vi "Actor Core.vi"(8 "error in":errorcluster, 11 "Rigol DG822 UI in":refnum<class "Rigol DG822 UI.lvclass">) -> (0 "error out":errorcluster, 3 "Actor out":refnum<class "Actor.lvclass">)   [LabVIEW 2021, in "Rigol DG822 UI.lvlib" / "Rigol DG822 UI.lvclass"]
uses:
  Rigol DG822 UI.lvclass
  General/Files/lvlibp/Actor Framework.lvlibp/1abvi3w/vi.lib/ActorFramework/Actor/Actor.lvclass
  D:/LabVIEW/General/Files/lvlibp/Actor Framework.lvlibp/1abvi3w/vi.lib/ActorFramework/Actor/Actor.lvclass
  D:/LabVIEW/General/Files/lvlibp/Actors.lvlibp/Actors/Actors/Actors.lvclass
  lib/controls.llb/DataCluster.ctl
  lib/controls.llb/String Indicators Cluster.ctl
  lib/controls.llb/FT Controls Cluster.ctl
  Rigol DG822 UI.lvclass/Rigol DG822 UI.ctl
  <vilib>/Utility/miscctls.llb/LVPointTypeDef.ctl
  lib/controls.llb/WaveformExtCall.ctl
  lib/controls.llb/WaveformSelector.ctl
  lib/controls.llb/RDG822ExtCall.ctl
  lib/controls.llb/AllWaveformDataCluster.ctl
  <userlib>/_MGI/Application Control/MGI VI Reference/MGI Current VI's Reference.vi
  <userlib>/_MGI/Timing/MGI Wait/MGI Wait (U32).vi
  General/Files/lvlibp/Actors.lvlibp/Actors/Actors/Actors.lvclass
  General/Files/lvlibp/Tools.lvlibp
panel:
  out "Data":T1={"Freq"={"Freq"=1.0, "FreqUnit"=enum."kHz", "FreqUnitPrcs"=9.0}, "Period"={"Period"=1.0, "PeriodUnit"=enum."ms", "PeriodUnitPrcs"=7.0}, "Ampl"={"Ampl"=5.0, "AmplUnit"=enum."Vpp", "AmplUnitPrcs"=4.0}, "HighL"={"HighL"=2.5, "HighLUnit"=enum."V", "HighLUnitPrcs"=4.0}, "Offset"={"Offset"=0.0, "OffsetUnit"=enum."Vdc", "OffsetUnitPrcs"=4.0}, "LowL"={"LowL"=-2.5, "LowLUnit"=enum."V", "LowLUnitPrcs"=4.0}, "Phase"={"Phase"=0.0, "PhaseUnit"=enum."°", "PhaseUnitPrcs"=3.0}, "Duty"={"Duty"=50.0, "DutyUnit"=enum."%", "DutyUnitPrcs"=3.0}, "Width"={"Width"=500.0, "WidthUnit"=enum."us", "WidthUnitPrcs"=4.0}, "RisEdge"={"RisEdge"=10.0, "RisEdgeUnit"=enum."ns", "RisEdgeUnitPrcs"=1.0}, "FallEdge"={"FallEdge"=10.0, "FallEdgeUnit"=enum."ns", "FallEdgeUnitPrcs"=1.0}} {"RisEdge"."RisEdge" format="%.1f"; "RisEdge"."RisEdgeUnitPrcs" format="%#_1g"; "FallEdge"."FallEdge" format="%.1f"; "FallEdge"."FallEdgeUnitPrcs" format="%#_1g"; "Width"."Width" format="%.4g"; "Width"."WidthUnitPrcs" format="%#_1g"; "Duty"."Duty" format="%.3g"; "Duty"."DutyUnitPrcs" format="%#_1g"; "Phase"."Phase" format="%.3g"; "Phase"."PhaseUnitPrcs" format="%#_1g"; "LowL"."LowL" format="%.4g"; "LowL"."LowLUnitPrcs" format="%#_1g"; "Offset"."Offset" format="%.4g"; "Offset"."OffsetUnitPrcs" format="%#_1g"; "HighL"."HighL" format="%.4g"; "HighL"."HighLUnitPrcs" format="%#_1g"; "Ampl"."Ampl" format="%.4g"; "Ampl"."AmplUnitPrcs" format="%#_1g"; "Period"."Period" format="%.7g"; "Period"."PeriodUnitPrcs" format="%#_1g"; "Freq"."FreqUnitPrcs" format="%#_1g"; "Freq"."Freq" format="%.9g"}
  in  "Out2":bool
  in  "Out1":bool
  in  "Home":bool
  in  "Main Tab":enum32{"Menu", "Wf Conf", "UpdScreen"}(tab)=enum."Wf Conf"
  in  "Wf Selector":T2(radio)=enum."Sine"
  out "Screen":picture
  in  "Menu":bool
  # "УБРАТЬ SINE ИЗ COERCE VALUE"
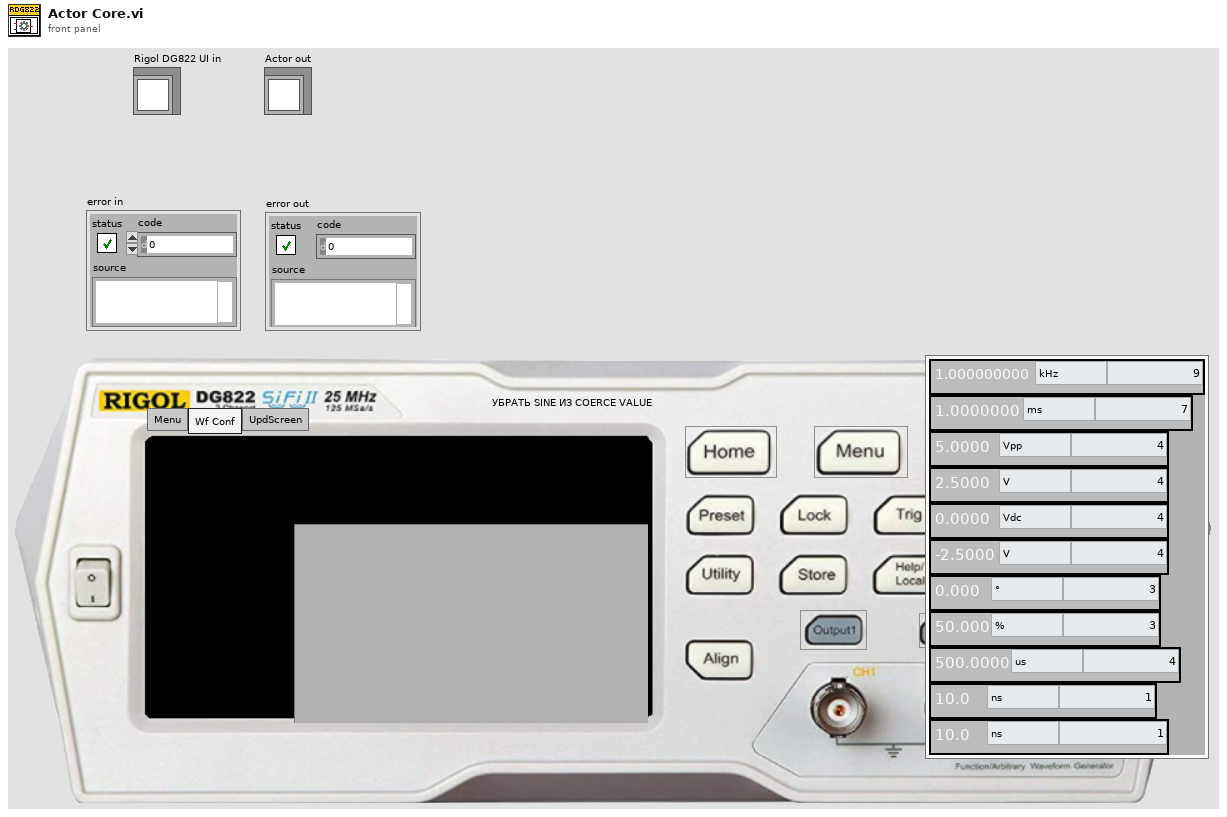
[diagram p1: front panel]
types:
  T1 = typedef "DataCluster.ctl" = cluster{"Freq":cluster{"Freq":dbl, "FreqUnit":enum32{"No Selection", "MHz", "kHz", "Hz", "mHz", "uHz"}, "FreqUnitPrcs":dbl}, "Period":cluster{"Period":dbl, "PeriodUnit":enum32{"No Selection", "s", "ms", "us", "ns"}, "PeriodUnitPrcs":dbl}, "Ampl":cluster{"Ampl":dbl, "AmplUnit":enum32{"No Selection", "Vpp", "mVpp"}, "AmplUnitPrcs":dbl}, "HighL":cluster{"HighL":dbl, "HighLUnit":enum32{"No Selection", "V", "mV"}, "HighLUnitPrcs":dbl}, "Offset":cluster{"Offset":dbl, "OffsetUnit":enum32{"No Selection", "Vdc", "mVdc"}, "OffsetUnitPrcs":dbl}, "LowL":cluster{"LowL":dbl, "LowLUnit":enum32{"No Selection", "V", "mV"}, "LowLUnitPrcs":dbl}, "Phase":cluster{"Phase":dbl, "PhaseUnit":enum32{"°"}, "PhaseUnitPrcs":dbl}, "Duty":cluster{"Duty":dbl, "DutyUnit":enum32{"%"}, "DutyUnitPrcs":dbl}, "Width":cluster{"Width":dbl, "WidthUnit":enum32{"No Selection", "s", "ms", "us", "ns"}, "WidthUnitPrcs":dbl}, "RisEdge":cluster{"RisEdge":dbl, "RisEdgeUnit":enum32{"No Selection", "s", "ms", "us", "ns"}, "RisEdgeUnitPrcs":dbl}, "FallEdge":cluster{"FallEdge":dbl, "FallEdgeUnit":enum32{"No Selection", "s", "ms", "us", "ns"}, "FallEdgeUnitPrcs":dbl}}
  T2 = enum32{"No Selection", "Sine", "Square", "Ramp", "Pulse", "Noise", "DC"}
  T3 = typedef "String Indicators Cluster.ctl" = cluster{"Freq-Period":string, "Ampl-HighL":string, "Offset-LowL":string, "Phase":string, "Duty-Width":string, "RisEdge":string, "FallEdge":string}
  T4 = typedef "FT Controls Cluster.ctl" = cluster{"Freq/Period":bool, "Ampl/HighL":bool, "Offset/LowL":bool, "Duty/Width":bool}
  T5 = cluster{"Name":string, "Prelaunch data":variant}[]
  T6 = cluster{"Actor names":string[], "VI Ref":refnum<vi>[], "Nested actors":refnum<class "Message Enqueuer.lvclass">[]}
  T7 = typedef "WaveformExtCall.ctl" = enum16{"Freq", "Period", "Ampl", "HighL", "Offset", "LowL", "Phase", "Duty", "Width", "RisEdge", "FallEdge", "Home", "InitData"}
  T8 = typedef "WaveformSelector.ctl" = enum32{"No Selection", "Sine", "Square", "Ramp", "Pulse", "Noise", "DC"}
  T9 = typedef "RDG822ExtCall.ctl" = enum16{"Get Data"}
  T10 = typedef "AllWaveformDataCluster.ctl" = cluster{"Data":T1, "F/T Ctrls":T4, "String Indcs":T3}
  T11 = typedef "LVPointTypeDef.ctl" = cluster{"Horizontal":i16, "Vertical":i16}
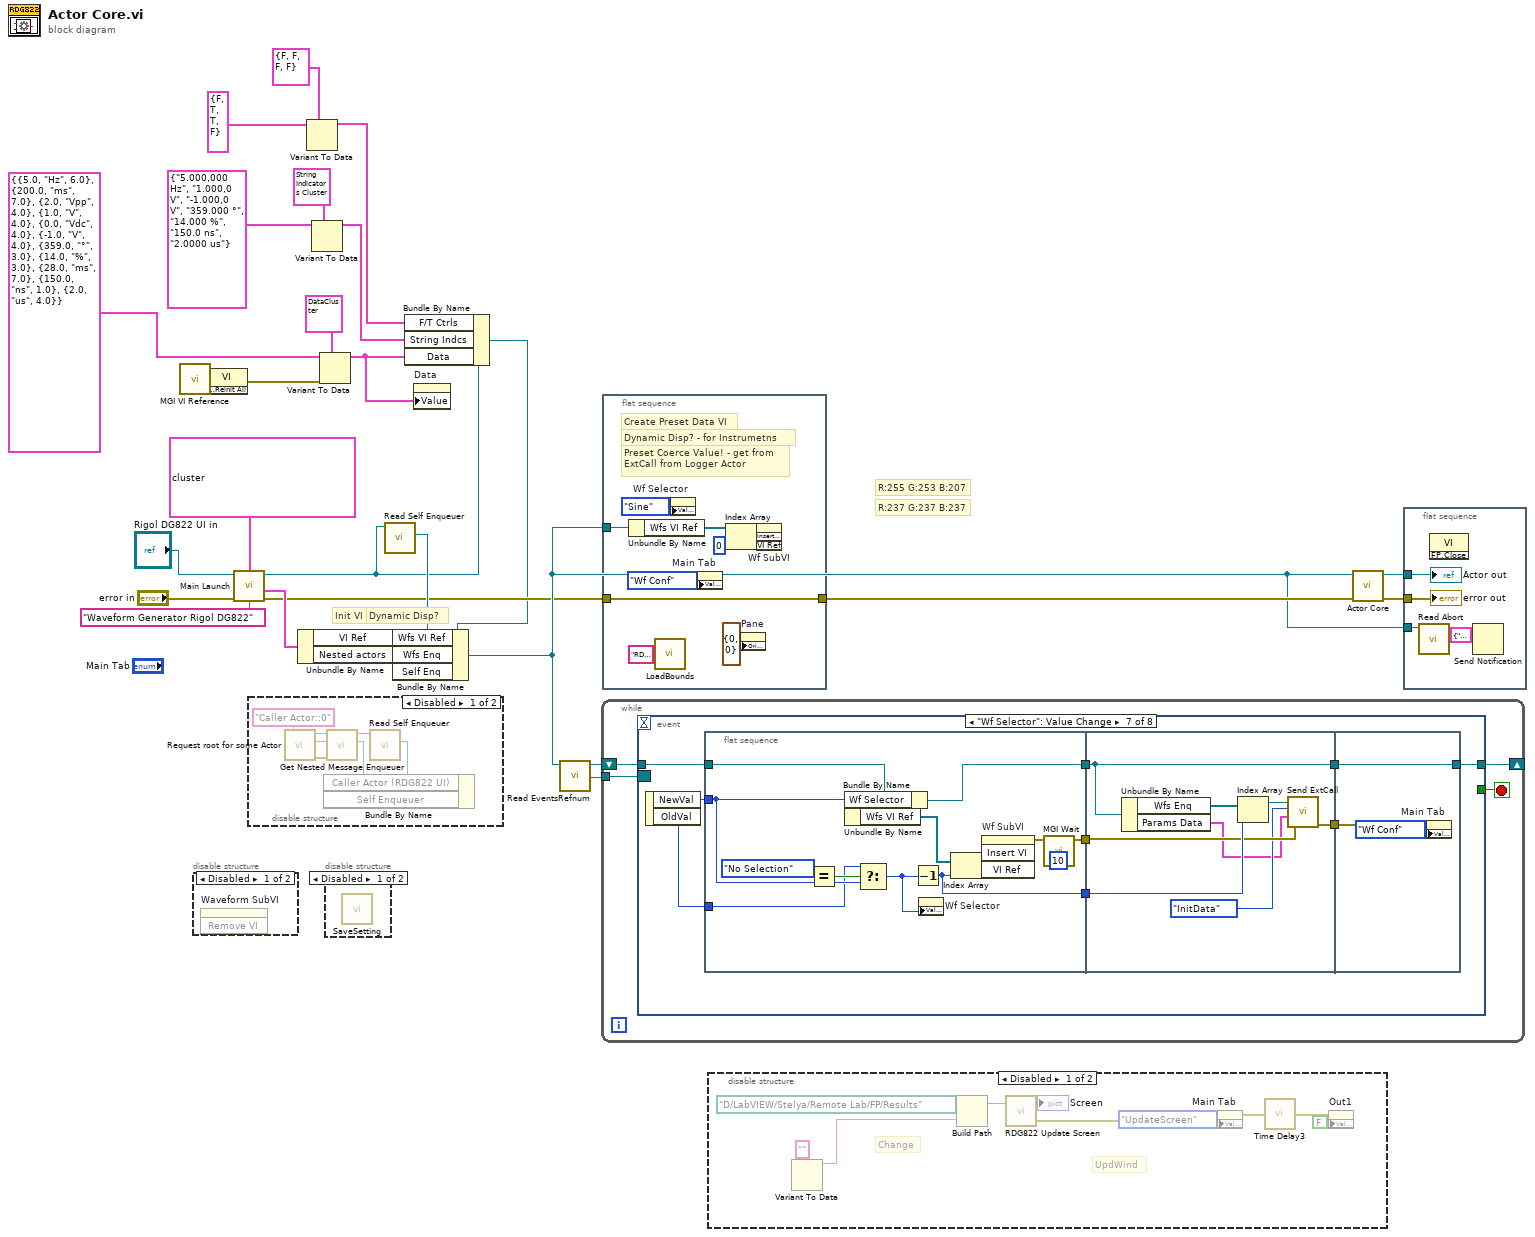
[diagram p0: block diagram]
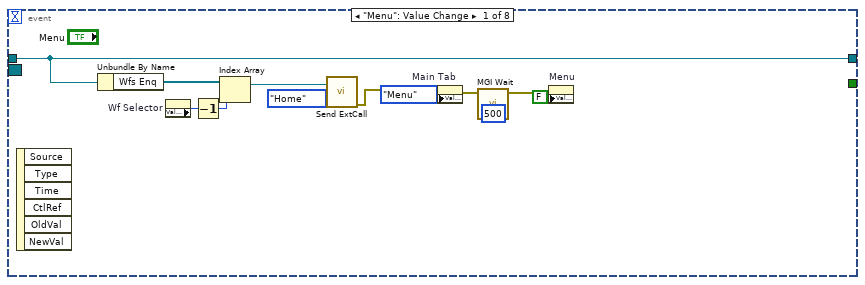
[diagram p5: hidden frame]
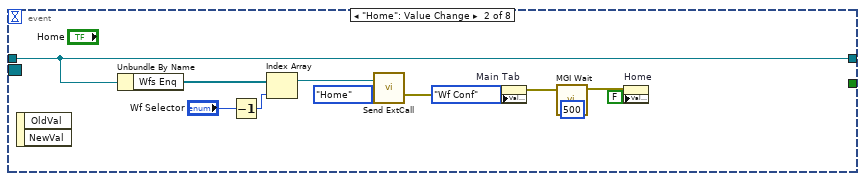
[diagram p6: hidden frame]
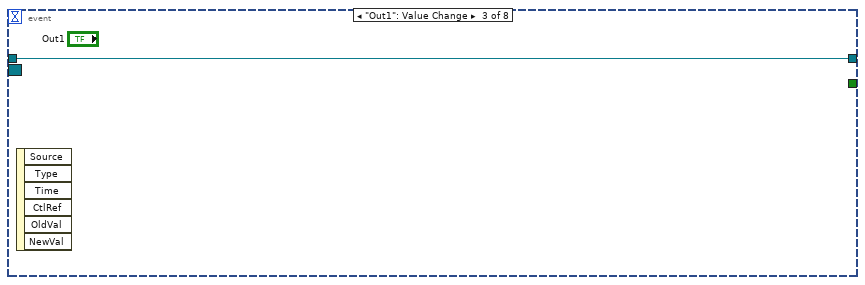
[diagram p7: hidden frame]
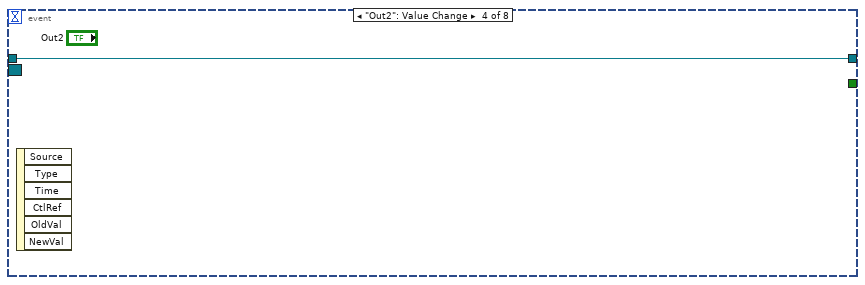
[diagram p8: hidden frame]
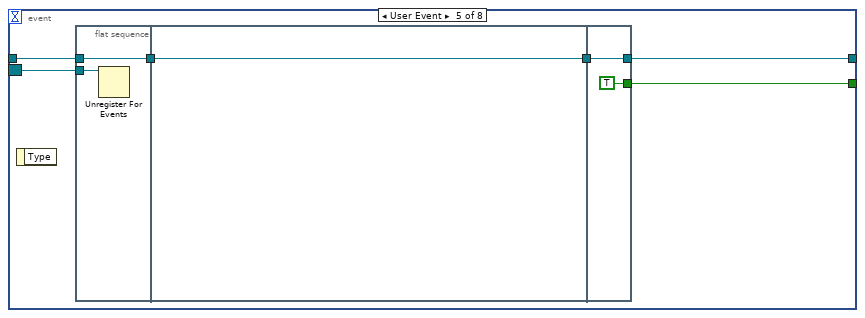
[diagram p9: hidden frame]
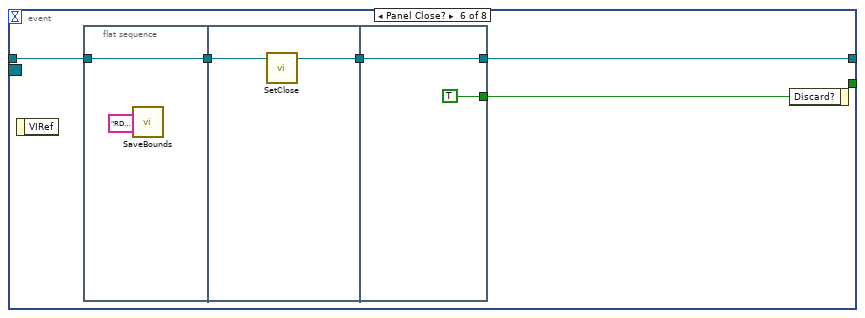
[diagram p10: hidden frame]
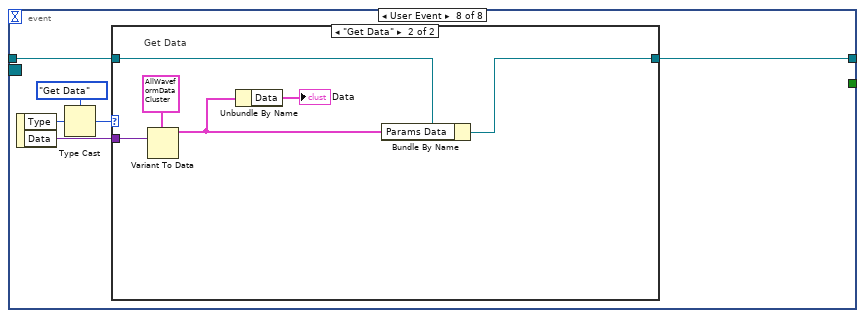
[diagram p11: hidden frame]
diagram:
  # "R:237 G:237 B:237"
  # "R:255 G:253 B:207"
  # "Dynamic Disp?"
  # "Init VI"
  n1 = call-poly <userlib>:"MGI VI Reference.vi"() -> ("Current VI's Reference"=w7:refnum<vi>)  [unwired: 1 in]
  n2 = disable-structure shown="Disabled" {
    frame Disabled {
      n3 = invoke on="Waveform SubVI" class="SubPnl" method="Remove VI"() -> ()  [unwired: 3 in, 3 out]
    }
    frame Enabled {
    }
  }
  n4 = invoke class="VI" method="Default Vals.Reinit All"(reference=w7) -> (error out=w6:errorcluster)  [unwired: 2 in, 2 out]
  n5 = call "Main Launch.vi"("Window Title"="Waveform Generator Rigol DG822", "Nested Actor names without extention"=T5 [{"Name"="Rigol DG822 Sine", "Prelaunch data"=variant}, {"Name"="Rigol DG822 Square", "Prelaunch data"=variant}, {"Name"="Rigol DG822 Pulse", "Prelaunch data"=variant}], "error in (no error)"="error in", "Actors in"="Rigol DG822 UI in") -> ("error out"=w9:errorcluster, "All VI Ref"=w20:T6, "Actors out"=w14:refnum<class "Rigol DG822 UI.lvclass">)  [unwired: 4 in, 1 out]
  n6 = disable-structure shown="Disabled" {
    frame Disabled {
      w29 = "Caller Actor::0" ("Actor Name")
      n7 = call "Request root for some Actor.vi"("Actor Name"=w29) -> ("error out"=w31:errorcluster, "Actors out"=w32:refnum<class "Actors.lvclass">)  [unwired: 9 in]
      n8 = call "Get Nested Message Enqueuer.vi"("Actor name ()"=w29, "error in (no error)"=w31, "Actors in"=w32) -> ("Message Enqueuer"=w30:refnum<class "Message Enqueuer.lvclass">, "Actors out"=w34:refnum<class "Actors.lvclass">)  [unwired: 4 in, 3 out]
      n9 = call "Read Self Enqueuer.vi"("Actor"=w34) -> ("Self Enqueuer"=w33:refnum<class "Message Enqueuer.lvclass">)  [unwired: 10 in]
      n10 = Bundle By Name("Caller Actor (RDG822 UI)"=w30, "Self Enqueuer"=w33) -> ()  [unwired: 1 in, 1 out]
    }
    frame Enabled {
    }
  }
  n11 = Unbundle By Name(w20) -> ("VI Ref"=w19:refnum<vi>[], "Nested actors"=w17:refnum<class "Message Enqueuer.lvclass">[])
  n12 = Variant To Data(type=T4 {"Freq/Period"=FALSE, "Ampl/HighL"=FALSE, "Offset/LowL"=FALSE, "Duty/Width"=FALSE} ("F/T Ctrls"), Variant=T4 {"Freq/Period"=FALSE, "Ampl/HighL"=TRUE, "Offset/LowL"=TRUE, "Duty/Width"=FALSE} ("F/T Ctrls")) -> (data=w12:T4)  [unwired: 1 in, 1 out]
  n13 = Variant To Data(type=T3 {"Freq-Period"="1.000,000,000 kHz", "Ampl-HighL"="5.000,0 Vpp", "Offset-LowL"="0.000,0 Vdc", "Phase"="0.000 °", "Duty-Width"="50.000 %", "RisEdge"="10.0 ns", "FallEdge"="10.0 ns"} ("String Indcs"), Variant=T3 {"Freq-Period"="5.000,000 Hz", "Ampl-HighL"="1.000,0 V", "Offset-LowL"="-1.000,0 V", "Phase"="359.000 °", "Duty-Width"="14.000 %", "RisEdge"="150.0 ns", "FallEdge"="2.0000 us"} ("String Indcs")) -> (data=w13:T3)  [unwired: 1 in, 1 out]
  n14 = Variant To Data(error in=w6, type=T1 {"Freq"={"Freq"=1.0, "FreqUnit"=enum."kHz", "FreqUnitPrcs"=9.0}, "Period"={"Period"=1.0, "PeriodUnit"=enum."ms", "PeriodUnitPrcs"=7.0}, "Ampl"={"Ampl"=5.0, "AmplUnit"=enum."Vpp", "AmplUnitPrcs"=4.0}, "HighL"={"HighL"=2.5, "HighLUnit"=enum."V", "HighLUnitPrcs"=4.0}, "Offset"={"Offset"=0.0, "OffsetUnit"=enum."Vdc", "OffsetUnitPrcs"=4.0}, "LowL"={"LowL"=-2.5, "LowLUnit"=enum."V", "LowLUnitPrcs"=4.0}, "Phase"={"Phase"=0.0, "PhaseUnit"=enum."°", "PhaseUnitPrcs"=3.0}, "Duty"={"Duty"=50.0, "DutyUnit"=enum."%", "DutyUnitPrcs"=3.0}, "Width"={"Width"=500.0, "WidthUnit"=enum."us", "WidthUnitPrcs"=4.0}, "RisEdge"={"RisEdge"=10.0, "RisEdgeUnit"=enum."ns", "RisEdgeUnitPrcs"=1.0}, "FallEdge"={"FallEdge"=10.0, "FallEdgeUnit"=enum."ns", "FallEdgeUnitPrcs"=1.0}} ("Data Cluster"), Variant=T1 {"Freq"={"Freq"=5.0, "FreqUnit"=enum."Hz", "FreqUnitPrcs"=6.0}, "Period"={"Period"=200.0, "PeriodUnit"=enum."ms", "PeriodUnitPrcs"=7.0}, "Ampl"={"Ampl"=2.0, "AmplUnit"=enum."Vpp", "AmplUnitPrcs"=4.0}, "HighL"={"HighL"=1.0, "HighLUnit"=enum."V", "HighLUnitPrcs"=4.0}, "Offset"={"Offset"=0.0, "OffsetUnit"=enum."Vdc", "OffsetUnitPrcs"=4.0}, "LowL"={"LowL"=-1.0, "LowLUnit"=enum."V", "LowLUnitPrcs"=4.0}, "Phase"={"Phase"=359.0, "PhaseUnit"=enum."°", "PhaseUnitPrcs"=3.0}, "Duty"={"Duty"=14.0, "DutyUnit"=enum."%", "DutyUnitPrcs"=3.0}, "Width"={"Width"=28.0, "WidthUnit"=enum."ms", "WidthUnitPrcs"=7.0}, "RisEdge"={"RisEdge"=150.0, "RisEdgeUnit"=enum."ns", "RisEdgeUnitPrcs"=1.0}, "FallEdge"={"FallEdge"=2.0, "FallEdgeUnit"=enum."us", "FallEdgeUnitPrcs"=4.0}} ("data")) -> (data=w10:T1)  [unwired: 1 out]
  n15 = disable-structure shown="Disabled" {
    frame Disabled {
      n16 = call "SaveSetting.vi"() -> ()  [unwired: 10 in, 2 out]
    }
    frame Enabled {
    }
  }
  n17 = call "Read Self Enqueuer.vi"("Actor"=w14) -> ("Self Enqueuer"=w15:refnum<class "Message Enqueuer.lvclass">)  [unwired: 10 in]
  n18 = Bundle By Name(cluster=w14, "F/T Ctrls"=w12, "String Indcs"=w13, "Data"=w10) -> (w8:refnum<class "Rigol DG822 UI.lvclass">)
  n19 = Bundle By Name(cluster=w8, "Wfs VI Ref"=w19, "Wfs Enq"=w17, "Self Enq"=w15) -> (w16:refnum<class "Rigol DG822 UI.lvclass">)
  n20 = property on="Data" class="Clust (strict)"("Value"=w10) -> ()  [unwired: 2 in, 2 out]
  n21 = call "Read EventsRefnum.vi"("Actors in"=w16) -> ("EventsRefnum"=w22:refnum<event-registration>, "Actors out"=w21:refnum<class "Rigol DG822 UI.lvclass">)  [unwired: 9 in]
  n22 = while {
    tunnel: w22 -> [w38]
    shift-right: [w36] -> _
    shift-left: w21 -> [w37]
    stop <- w35 stop-if-true
    n23 = event shown="[6] \"Wf Selector\": Value Change" {
      selector: w38 -> [_ _ _ _ w69 _ _ _]
      dyn-events: _ -> [_ _ _ _ _ _ _ _]
      timeout: _ -> [_ _ _ _ _ _ _ _]
      tunnel: w37 -> [w46 w61 w63 w64 w67 w79 w94 w125]
      tunnel: [w46 w61 w63 w64 w65 w76 w95 w124] -> w36
      tunnel: [_ _ _ _ w70 _ _ _] -> w35
      event "Menu": Value Change {
        n24 = event-data() -> ()  [unwired: 1 in, 6 out]
        n25 = Unbundle By Name(w46) -> ("Wfs Enq"=w45:refnum<class "Message Enqueuer.lvclass">[])
        n26 = property on="Wf Selector" class="RadioBtnsControl (strict)"() -> ("Value"=w44:T2)  [unwired: 2 in, 2 out]
        n27 = Decrement(x=w44) -> (x-1=w43:T2)
        n28 = Index Array(array=w45, index=w43) -> (element=w49:refnum<class "Message Enqueuer.lvclass">)
        n29 = call "Send ExtCall.vi"("Tag"=WaveformExtCall."Home" ("SineExtCall"), "Message Enqueuer"=w49) -> ("error out"=w47:errorcluster)  [unwired: 6 in, 3 out]
        n30 = property on="Main Tab" class="TabCtl (strict)"(error in=w47, "Value"=enum32{"Menu", "Wf Conf", "UpdScreen"}."Menu" ("Main Tab")) -> (error out=w41:errorcluster)  [unwired: 1 in, 1 out]
        n31 = call-poly <userlib>:"MGI Wait.vi"("ms"=u32 500, "Error In"=w41) -> ("Error Out"=w39:errorcluster)  [unwired: 5 in]
        n32 = property on="Menu" class="Bool (strict)"(error in=w39, "Value"=FALSE ("Menu")) -> ()  [unwired: 1 in, 2 out]
      }
      event "Home": Value Change {
        n33 = event-data() -> ()  [unwired: 1 in, 2 out]
        n34 = Unbundle By Name(w61) -> ("Wfs Enq"=w58:refnum<class "Message Enqueuer.lvclass">[])
        n35 = Decrement(x="Wf Selector") -> (x-1=w59:T2)
        n36 = Index Array(array=w58, index=w59) -> (element=w57:refnum<class "Message Enqueuer.lvclass">)
        n37 = call "Send ExtCall.vi"("Tag"=WaveformExtCall."Home" ("SineExtCall"), "Message Enqueuer"=w57) -> ("error out"=w60:errorcluster)  [unwired: 6 in, 3 out]
        n38 = property on="Main Tab" class="TabCtl (strict)"(error in=w60, "Value"=enum32{"Menu", "Wf Conf", "UpdScreen"}."Wf Conf" ("Main Tab")) -> (error out=w53:errorcluster)  [unwired: 1 in, 1 out]
        n39 = call-poly <userlib>:"MGI Wait.vi"("ms"=u32 500, "Error In"=w53) -> ("Error Out"=w52:errorcluster)  [unwired: 5 in]
        n40 = property on="Home" class="Bool (strict)"(error in=w52, "Value"=FALSE ("Menu")) -> ()  [unwired: 1 in, 2 out]
      }
      event "Out1": Value Change {
        n41 = event-data() -> ()  [unwired: 1 in, 6 out]
      }
      event "Out2": Value Change {
        n42 = event-data() -> ()  [unwired: 1 in, 6 out]
      }
      event User Event {
        n43 = event-data() -> ()  [unwired: 1 in, 1 out]
        n44 = flat-sequence {
          tunnel: w69 -> [w72]
          tunnel: [w71] -> w68
          tunnel: w67 -> [w71]
          tunnel: w68 -> [w73]
          tunnel: [w73] -> w66
          tunnel: [TRUE] -> w70
          tunnel: w66 -> [w74]
          tunnel: [w74] -> w65
          frame #0 {
            n45 = Unregister For Events(event registration refnum=w72) -> ()  [unwired: 1 in, 1 out]
          }
          frame #1 {
          }
          frame #2 {
          }
        }
      }
      event Panel Close? {
        n46 = event-data() -> ()  [unwired: 1 in, 1 out]
        n47 = flat-sequence {
          tunnel: w79 -> [w82]
          tunnel: [w82] -> w78
          tunnel: w78 -> [w84]
          tunnel: [w83] -> w77
          tunnel: [TRUE] -> w80
          tunnel: [w85] -> w76
          tunnel: w77 -> [w85]
          frame #0 {
            n48 = call "SaveBounds.vi"("SettingName"="RDG822UI.bounds") -> ()
          }
          frame #1 {
            n49 = call "SetClose.vi"("Actors in"=w84) -> ("Actors out"=w83:refnum<class "Rigol DG822 UI.lvclass">)  [unwired: 9 in, 1 out]
          }
          frame #2 {
          }
        }
        n50 = event-data("Discard?"=w80) -> ()  [unwired: 1 in, 1 out]
      }
      event "Wf Selector": Value Change {
        n51 = event-data() -> ("NewVal"=w93:T2, "OldVal"=w92:T2)  [unwired: 1 in]
        n52 = flat-sequence {
          tunnel: w94 -> [w107]
          tunnel: w93 -> [w101]
          tunnel: w92 -> [w100]
          tunnel: [w108] -> w91
          tunnel: [w97] -> w90
          tunnel: [w96] -> w88
          tunnel: w91 -> [w111]
          tunnel: w90 -> [w115]
          tunnel: [w113] -> w89
          tunnel: w88 -> [w112]
          tunnel: [w111] -> w87
          tunnel: [w119] -> w95
          tunnel: w89 -> [w117]
          tunnel: w87 -> [w119]
          frame #0 {
            n53 = Equal?(x=WaveformSelector."No Selection" ("NewVal"), y=w101) -> (x = y?=w103:bool)
            n54 = Bundle By Name(cluster=w107, "Wf Selector"=w101) -> (w108:refnum<class "Rigol DG822 UI.lvclass">)
            n55 = Unbundle By Name(w107) -> ("Wfs VI Ref"=w106:refnum<vi>[])
            n56 = Select(t=w100, s=w103, f=w101) -> (s? t:f=w99:T2)
            n57 = Decrement(x=w99) -> (x-1=w97:T2)
            n58 = property on="Wf Selector" class="RadioBtnsControl (strict)"("Value"=w99) -> ()  [unwired: 2 in, 2 out]
            n59 = Index Array(array=w106, index=w97) -> (element=w105:refnum<vi>)
            n60 = invoke on="Wf SubVI" class="SubPnl" method="Insert VI"("VI Ref"=w105) -> (error out=w104:errorcluster)  [unwired: 3 in, 3 out]
            n61 = call-poly <userlib>:"MGI Wait.vi"("ms"=u32 10, "Error In"=w104) -> ("Error Out"=w96:errorcluster)  [unwired: 5 in]
          }
          frame #1 {
            n62 = Unbundle By Name(w111) -> ("Wfs Enq"=w116:refnum<class "Message Enqueuer.lvclass">[], "Params Data"=w109:T10)
            n63 = Index Array(array=w116, index=w115) -> (element=w114:refnum<class "Message Enqueuer.lvclass">)
            n64 = call "Send ExtCall.vi"("error in (no error)"=w112, "Val"=w109, "Tag"=WaveformExtCall."InitData" ("SineExtCall"), "Message Enqueuer"=w114) -> ("error out"=w113:errorcluster)  [unwired: 4 in, 3 out]
          }
          frame #2 {
            n65 = property on="Main Tab" class="TabCtl (strict)"(error in=w117, "Value"=enum32{"Menu", "Wf Conf", "UpdScreen"}."Wf Conf" ("Main Tab")) -> ()  [unwired: 1 in, 2 out]
          }
        }
      }
      event User Event {
        n66 = event-data() -> ("Type"=w122:u16, "Data"=w123:variant)  [unwired: 1 in]
        n67 = Type Cast(type=RDG822ExtCall."Get Data", x=w122) -> (*(type *) &x=w121:T9)
        n68 = case shown="\"Get Data\"" w121 {
          tunnel: w125 -> [w126 w131]
          tunnel: [w126 w130] -> w124
          tunnel: w123 -> [_ w132]
          frame Default {
          }
          frame "Get Data" {
            # "Get Data"
            n69 = Variant To Data(type=T10 {"Data"={"Freq"={"Freq"=1.0, "FreqUnit"=enum."kHz", "FreqUnitPrcs"=9.0}, "Period"={"Period"=1.0, "PeriodUnit"=enum."ms", "PeriodUnitPrcs"=7.0}, "Ampl"={"Ampl"=5.0, "AmplUnit"=enum."Vpp", "AmplUnitPrcs"=4.0}, "HighL"={"HighL"=2.5, "HighLUnit"=enum."V", "HighLUnitPrcs"=4.0}, "Offset"={"Offset"=0.0, "OffsetUnit"=enum."Vdc", "OffsetUnitPrcs"=4.0}, "LowL"={"LowL"=-2.5, "LowLUnit"=enum."V", "LowLUnitPrcs"=4.0}, "Phase"={"Phase"=0.0, "PhaseUnit"=enum."°", "PhaseUnitPrcs"=3.0}, "Duty"={"Duty"=50.0, "DutyUnit"=enum."%", "DutyUnitPrcs"=3.0}, "Width"={"Width"=500.0, "WidthUnit"=enum."us", "WidthUnitPrcs"=4.0}, "RisEdge"={"RisEdge"=10.0, "RisEdgeUnit"=enum."ns", "RisEdgeUnitPrcs"=1.0}, "FallEdge"={"FallEdge"=10.0, "FallEdgeUnit"=enum."ns", "FallEdgeUnitPrcs"=1.0}}, "F/T Ctrls"={"Freq/Period"=FALSE, "Ampl/HighL"=FALSE, "Offset/LowL"=FALSE, "Duty/Width"=FALSE}, "String Indcs"={"Freq-Period"="1.000,000,000 kHz", "Ampl-HighL"="5.000,0 Vpp", "Offset-LowL"="0.000,0 Vdc", "Phase"="0.000 °", "Duty-Width"="50.000 %", "RisEdge"="10.0 ns", "FallEdge"="10.0 ns"}} ("Params Data"), Variant=w132) -> (data=w129:T10)  [unwired: 1 in, 1 out]
            n70 = Unbundle By Name(w129) -> ("Data"=→"Data":T1)
            n71 = Bundle By Name(cluster=w131, "Params Data"=w129) -> (w130:refnum<class "Rigol DG822 UI.lvclass">)
          }
        }
      }
    }
  }
  n72 = flat-sequence {
    tunnel: w9 -> [w140]
    tunnel: [w140] -> w23
    tunnel: w16 -> [w134]
    frame #0 {
      # "Preset Coerce Value! - get from\nExtCall from Logger Actor"
      # "Dynamic Disp? - for Instrumetns"
      # "Create Preset Data VI"
      n73 = Unbundle By Name(w134) -> ("Wfs VI Ref"=w138:refnum<vi>[])
      n74 = call "LoadBounds.vi"("SettingName"="RDG822UI.bounds") -> ()
      n75 = property on="Wf Selector" class="RadioBtnsControl (strict)"("Value"=T2."Sine" ("Wavefrom Selector")) -> ()  [unwired: 2 in, 2 out]
      n76 = property on="Main Tab" class="TabCtl (strict)"("Value"=enum32{"Menu", "Wf Conf", "UpdScreen"}."Wf Conf" ("Main Tab")) -> ()  [unwired: 2 in, 2 out]
      n77 = Index Array(array=w138, index=0) -> (element=w137:refnum<vi>)
      n78 = property on="Pane" class="Pane"("Origin"=T11 {"Horizontal"=0, "Vertical"=0}) -> ()  [unwired: 2 in, 2 out]
      n79 = invoke on="Wf SubVI" class="SubPnl" method="Insert VI"("VI Ref"=w137) -> ()  [unwired: 3 in, 4 out]
    }
  }
  n80 = disable-structure shown="Disabled" {
    frame Disabled {
      # "UpdWind"
      # "Change"
      n81 = Variant To Data(type="") -> (data=w151:string)  [unwired: 2 in, 1 out]
      n82 = Build Path(base path=path "D:/LabVIEW/Stelya/Remote Lab/FP/Results" ("Path to file"), name or relative path=w151) -> (appended path=w150:path)
      n83 = call "RDG822 Update Screen.vi"("Path to file"=w150) -> ("error out"=w149:errorcluster, "Screen"=→"Screen":picture)  [unwired: 9 in]
      n84 = property on="Main Tab" class="TabCtl (strict)"(error in=w149, "Value"=enum32{"Menu", "SignalConf", "UpdateScreen"}."UpdateScreen" ("Value (Signaling)")) -> (error out=w146:errorcluster)  [unwired: 1 in, 1 out]
      n85 = call "Time Delay3"("error in (no error)"=w146) -> ("error out"=w147:errorcluster)  [unwired: 10 in]
      n86 = property on="Out1" class="Bool (strict)"(error in=w147, "Value"=FALSE ("Menu")) -> ()  [unwired: 1 in, 2 out]
    }
    frame Enabled {
    }
  }
  n87 = call-parent "Actor Core.vi"("error in"=w23, "Actor in"=w16) -> ("error out"=w28:errorcluster, "Actor out"=w27:refnum<class "Actor.lvclass">)  [unwired: 8 in]
  n88 = flat-sequence {
    tunnel: w28 -> [w156]
    tunnel: w27 -> [w153]
    tunnel: w16 -> [w152]
    frame #0 {
      n89 = call "Read Abort.vi"("Actors in"=w152) -> ("AbortEvent"=w155:refnum<notifier>)  [unwired: 10 in]
      n90 = invoke class="VI" method="FP.Close"() -> ()  [unwired: 3 in, 3 out]
      n91 = Send Notification(notification=cluster{"Caller":string, "AnyValue":variant} {"Caller"="abort", "AnyValue"=variant}, notifier=w155) -> ()  [unwired: 1 in, 2 out]
      "error out" <- w156
      "Actor out" <- w153
    }
  }
